vi "E9_Semaforo_LocVar.vi"() -> ()   [LabVIEW 2020]
panel:
  out "R2":bool=TRUE
  out "A2":bool=TRUE
  out "V2":bool=TRUE
  out "R1":bool=TRUE
  out "A1":bool=TRUE
  out "V1":bool=TRUE
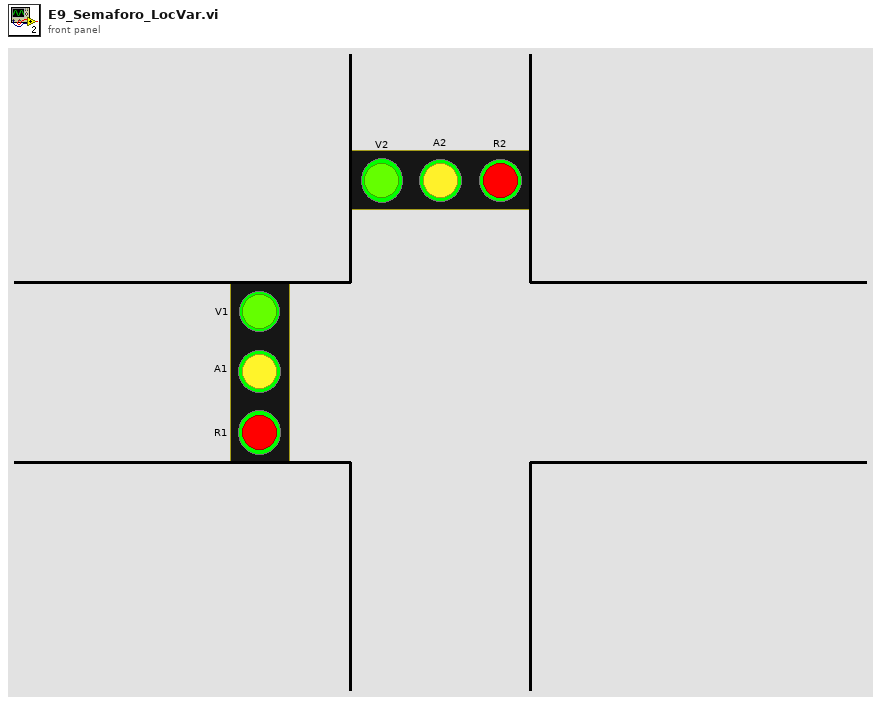
[diagram p1: front panel]
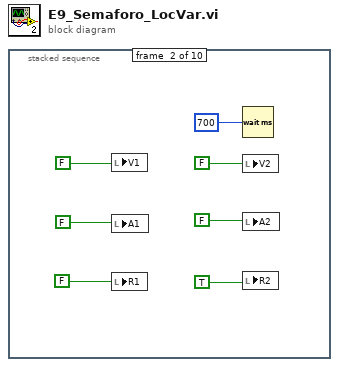
[diagram p0: block diagram]
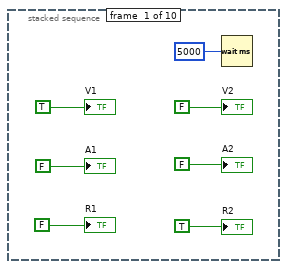
[diagram p2: hidden frame]
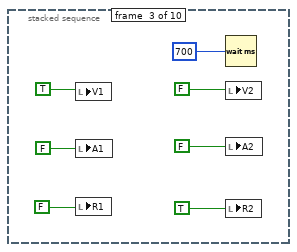
[diagram p3: hidden frame]
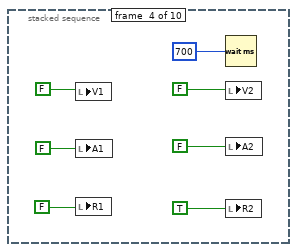
[diagram p4: hidden frame]
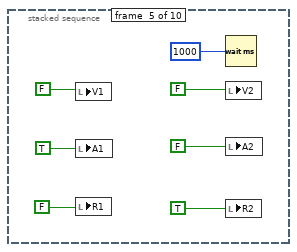
[diagram p5: hidden frame]
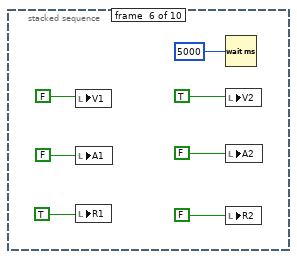
[diagram p6: hidden frame]
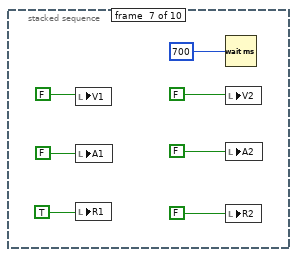
[diagram p7: hidden frame]
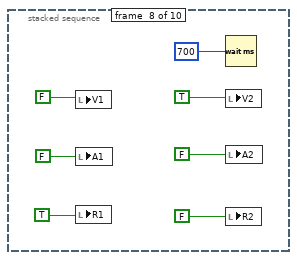
[diagram p8: hidden frame]
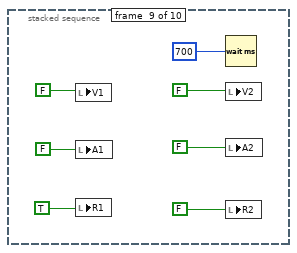
[diagram p9: hidden frame]
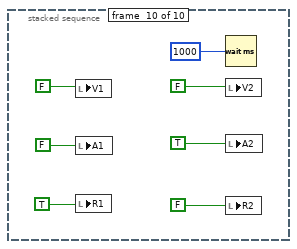
[diagram p10: hidden frame]
diagram:
  n1 = stacked-sequence {
    frame #0 {
      n2 = Wait (ms)(milliseconds to wait=u32 5000) -> ()  [unwired: 1 out]
      "V1" <- TRUE
      "A1" <- FALSE
      "R1" <- FALSE
      "V2" <- FALSE
      "A2" <- FALSE
      "R2" <- TRUE
    }
    frame #1 {
      n3 = local write "V1"(FALSE) -> ()
      n4 = local write "A1"(FALSE) -> ()
      n5 = local write "R1"(FALSE) -> ()
      n6 = Wait (ms)(milliseconds to wait=u32 700) -> ()  [unwired: 1 out]
      n7 = local write "V2"(FALSE) -> ()
      n8 = local write "A2"(FALSE) -> ()
      n9 = local write "R2"(TRUE) -> ()
    }
    frame #2 {
      n10 = local write "V1"(TRUE) -> ()
      n11 = local write "A1"(FALSE) -> ()
      n12 = local write "R1"(FALSE) -> ()
      n13 = Wait (ms)(milliseconds to wait=u32 700) -> ()  [unwired: 1 out]
      n14 = local write "V2"(FALSE) -> ()
      n15 = local write "A2"(FALSE) -> ()
      n16 = local write "R2"(TRUE) -> ()
    }
    frame #3 {
      n17 = local write "V1"(FALSE) -> ()
      n18 = local write "A1"(FALSE) -> ()
      n19 = local write "R1"(FALSE) -> ()
      n20 = Wait (ms)(milliseconds to wait=u32 700) -> ()  [unwired: 1 out]
      n21 = local write "V2"(FALSE) -> ()
      n22 = local write "A2"(FALSE) -> ()
      n23 = local write "R2"(TRUE) -> ()
    }
    frame #4 {
      n24 = local write "V1"(FALSE) -> ()
      n25 = local write "A1"(TRUE) -> ()
      n26 = local write "R1"(FALSE) -> ()
      n27 = Wait (ms)(milliseconds to wait=u32 1000) -> ()  [unwired: 1 out]
      n28 = local write "V2"(FALSE) -> ()
      n29 = local write "A2"(FALSE) -> ()
      n30 = local write "R2"(TRUE) -> ()
    }
    frame #5 {
      n31 = local write "V1"(FALSE) -> ()
      n32 = local write "A1"(FALSE) -> ()
      n33 = local write "R1"(TRUE) -> ()
      n34 = Wait (ms)(milliseconds to wait=u32 5000) -> ()  [unwired: 1 out]
      n35 = local write "V2"(TRUE) -> ()
      n36 = local write "A2"(FALSE) -> ()
      n37 = local write "R2"(FALSE) -> ()
    }
    frame #6 {
      n38 = local write "V1"(FALSE) -> ()
      n39 = local write "A1"(FALSE) -> ()
      n40 = local write "R1"(TRUE) -> ()
      n41 = Wait (ms)(milliseconds to wait=u32 700) -> ()  [unwired: 1 out]
      n42 = local write "V2"(FALSE) -> ()
      n43 = local write "A2"(FALSE) -> ()
      n44 = local write "R2"(FALSE) -> ()
    }
    frame #7 {
      n45 = local write "V1"(FALSE) -> ()
      n46 = local write "A1"(FALSE) -> ()
      n47 = local write "R1"(TRUE) -> ()
      n48 = Wait (ms)(milliseconds to wait=u32 700) -> ()  [unwired: 1 out]
      n49 = local write "V2"(TRUE) -> ()
      n50 = local write "A2"(FALSE) -> ()
      n51 = local write "R2"(FALSE) -> ()
    }
    frame #8 {
      n52 = local write "V1"(FALSE) -> ()
      n53 = local write "A1"(FALSE) -> ()
      n54 = local write "R1"(TRUE) -> ()
      n55 = Wait (ms)(milliseconds to wait=u32 700) -> ()  [unwired: 1 out]
      n56 = local write "V2"(FALSE) -> ()
      n57 = local write "A2"(FALSE) -> ()
      n58 = local write "R2"(FALSE) -> ()
    }
    frame #9 {
      n59 = local write "V1"(FALSE) -> ()
      n60 = local write "A1"(FALSE) -> ()
      n61 = local write "R1"(TRUE) -> ()
      n62 = Wait (ms)(milliseconds to wait=u32 1000) -> ()  [unwired: 1 out]
      n63 = local write "V2"(FALSE) -> ()
      n64 = local write "A2"(TRUE) -> ()
      n65 = local write "R2"(FALSE) -> ()
    }
  }
